vi "FTW-Router-Construct.vi"(5 "Address":string, 11 "error in":errorcluster) -> (4 "FTW-Router Out":refnum<class "FTW-Router.lvclass">, 6 "Actual Address":string, 10 "Event Registration Refnum":refnum<event-registration>, 15 "error out":errorcluster)   [LabVIEW 2013, in "FTW-Router.lvclass"]
uses:
  FTW-Router.lvclass
  Message/Request/FTW-Message-IncomingRequest.lvclass
  Listener/FTW-Listener.lvclass
  FTW-Router.lvclass/FTW-Router.ctl
  Ether/FTW-Ether.lvclass
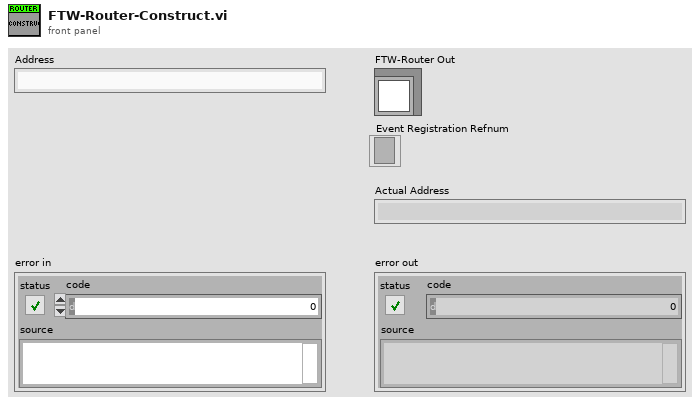
[diagram p1: front panel]
types:
  T1 = typedef "FTW-Ether.lvclass/FTW-Ether-MessageTransportScheme.ctl" = enum16{"LabVIEW Queues (lvq://)", "TCP (tcp://)", "LabVIEW Network Streams (lvns://)"}
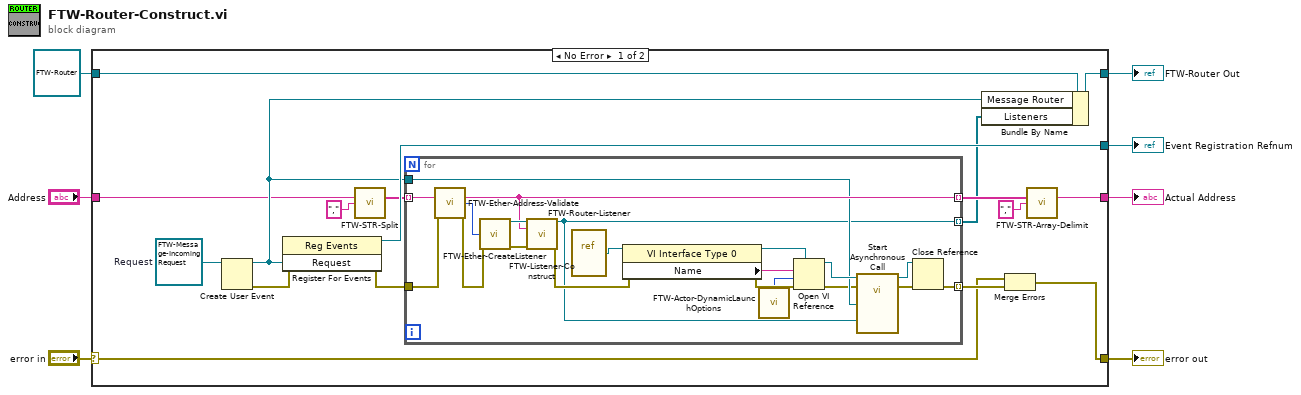
[diagram p0: block diagram]
diagram:
  n1 = case shown="No Error" "error in" {
    selector: "error in" -> [w9 w46]
    tunnel: [w11 w46] -> w6
    tunnel: [w24 w45] -> w5
    tunnel: [w23 _] -> w3
    tunnel: "Address" -> [w15 _]
    tunnel: [w13 _] -> w2
    tunnel: refnum<class "FTW-Router.lvclass"> refnum ("LVmsg_Router.lvclass") -> [w19 w45]
    frame No Error {
      w22 = refnum<class "FTW-Message-IncomingRequest.lvclass"> refnum  # Request
      n2 = Create User Event(user event datatype=w22) -> (user event=w20:refnum<user-event>, error out=w17:errorcluster)  [unwired: 1 in]
      n3 = register-events(error in=w17, w20) -> (reference out=w23:refnum<event-registration>, error out=w10:errorcluster)  [unwired: 1 in]
      n4 = call "FTW-STR-Split.vi"("Delimited String"=w15, "Delimiter"=",") -> ("Array of Strings"=w8:string[])  [unwired: 13 in]
      n5 = for {
        tunnel: [w32] -> w21 mode=indexing
        tunnel: w20 -> [w31]
        tunnel: w10 -> [w29]
        tunnel: [w27] -> w18 mode=indexing
        tunnel: w8 -> [w26] mode=indexing
        tunnel: [w25] -> w14 mode=indexing
        n6 = call "FTW-Ether-Address-Validate.vi"("Address"=w26, "error in"=w29) -> ("Sanitized Address"=w32:string, "Message Transport Scheme"=w33:T1, "error out"=w34:errorcluster)  [unwired: 11 in]
        n7 = call "FTW-Ether-CreateListener.vi"("Message Transport Scheme"=w33, "error in"=w34) -> ("FTW-Listener"=w36:refnum<class "FTW-Listener.lvclass">, "error out"=w35:errorcluster)  [unwired: 12 in]
        n8 = call-dynamic "FTW-Listener-Construct.vi"("Gmsg_Listener In"=w36, "Address"=w32, "error in"=w35) -> ("Gmsg_Listener Out"=w25:refnum<class "FTW-Listener.lvclass">, "error out"=w30:errorcluster)  [unwired: 11 in]
        n9 = vi-ref "FTW-Router-Listener.vi"() -> (w44:refnum<vi>)
        n10 = property class="VI Interface Type 0"(reference=w44, error in=w30) -> (reference out=w40:refnum<vi>, error out=w43:errorcluster, "Name"=w42:string)
        n11 = call "FTW-Actor-DynamicLaunchOptions.vi"() -> ("Open VI Ref Options"=w41:i32)
        n12 = Open VI Reference(type specifier VI Refnum (for type only)=w40, vi path=w42, options=w41, error in (no error)=w43) -> (vi reference=w38:refnum<vi>, error out=w28:errorcluster)  [unwired: 2 in]
        n13 = call-by-ref "Start Asynchronous Call"(reference=w38, error in=w28, "Listener"=w25, "Message Handler"=w31) -> (reference out=w37:refnum<vi>, error out=w39:errorcluster)  [unwired: 1 in]
        n14 = Close Reference(reference=w37, error in (no error)=w39) -> (error out=w27:errorcluster)
      }
      n15 = Bundle By Name(cluster=w19, "Message Router"=w20, "Listeners"=w14) -> (w24:refnum<class "FTW-Router.lvclass">)
      n16 = Merge Errors(w9, w18) -> (w11:errorcluster)
      n17 = call "FTW-STR-Array-Delimit.vi"("Array of Strings"=w21, "Delimiter"=",") -> ("Delimited String"=w13:string)  [unwired: 13 in]
    }
    frame Error {
    }
  }
  "FTW-Router Out" <- w5
  "error out" <- w6
  "Event Registration Refnum" <- w3
  "Actual Address" <- w2
